vi "Read All DAQChannels.vi"(8 "error in (no error)":errorcluster, 11 "IODevConfig in":refnum<class "IODevConfig.lvclass">) -> (0 "error out":errorcluster, 2 "All DAQChannels":tag[](array[tag]), 3 "IODevConfig out":refnum<class "IODevConfig.lvclass">)   [LabVIEW 2015, in "IODevConfig.lvclass"]
uses:
  IODevConfig.lvclass
  IODevConfig.lvclass/IODevConfig.ctl
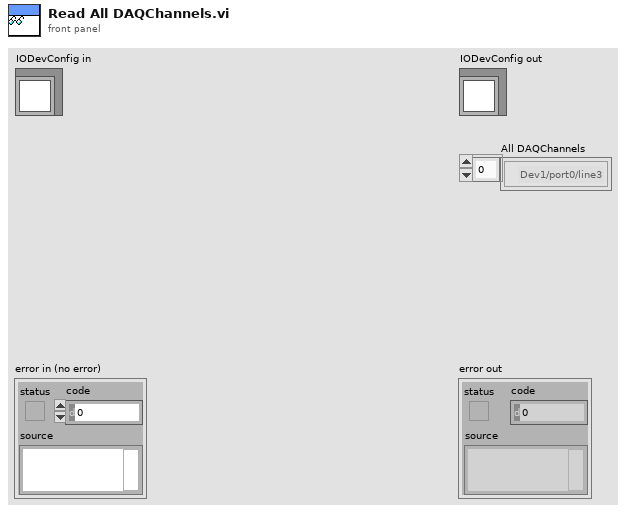
[diagram p1: front panel]
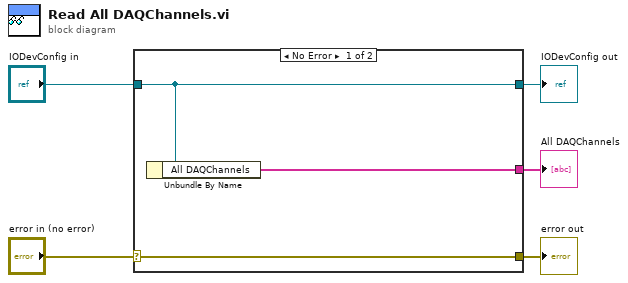
[diagram p0: block diagram]
diagram:
  n1 = case shown="No Error" "error in (no error)" {
    selector: "error in (no error)" -> [w8 w9]
    tunnel: [w8 w9] -> w4
    tunnel: [w7 w10] -> w2
    tunnel: "IODevConfig in" -> [w7 w10]
    tunnel: [w6 _] -> w1
    frame No Error {
      n2 = Unbundle By Name(w7) -> ("All DAQChannels"=w6:tag[])
    }
    frame Error {
    }
  }
  "error out" <- w4
  "IODevConfig out" <- w2
  "All DAQChannels" <- w1
